vi "MFC.vi"() -> ()   [LabVIEW 2016]
uses:
  controls/UI Data.ctl
  Settings/Settings.ctl
  Logging/Logging Configuration.ctl
  Acquisition/Hardware Configuration.ctl
  controls/UI State.ctl
  support/Message Queue/Enqueue Message (Single).vi
  support/Message Queue/Enqueue Message (Array).vi
  <vilib>/Utility/error.llb/Error Cluster From Error Code.vi
  <vilib>/ErrorRing/Error Ring.xnode
  Settings/Settings.lvlib
  support/Message Queue/Message Queue.lvlib
  Settings/Settings Dialog.vi
  support/User Event - Stop/User Event - Stop.lvlib
  Logging/Logging.lvlib
  Acquisition/Acquisition.lvlib
panel:
  in  "Reset":bool
  out "Total":dbl
  out "R.P":dbl
  in  "S.P.":dbl
  in  "Control":enum32{"1", "2", "4"}(radio)
  in  "Control Mode":T1(radio)
  out "Data":waveform(dbl)[](graph)
  out "2":dbl(knob) caption="总流量" scale=0.0..100.0
  out "流量设定":cluster{dbl, dbl}(knob) scale=0.0..1.0
  in  "Exit":bool
  in  "Stop":bool
  in  "Settings":bool
  in  "Start":bool
  in  "Show Mode":T1(radio)
  out "Status":string
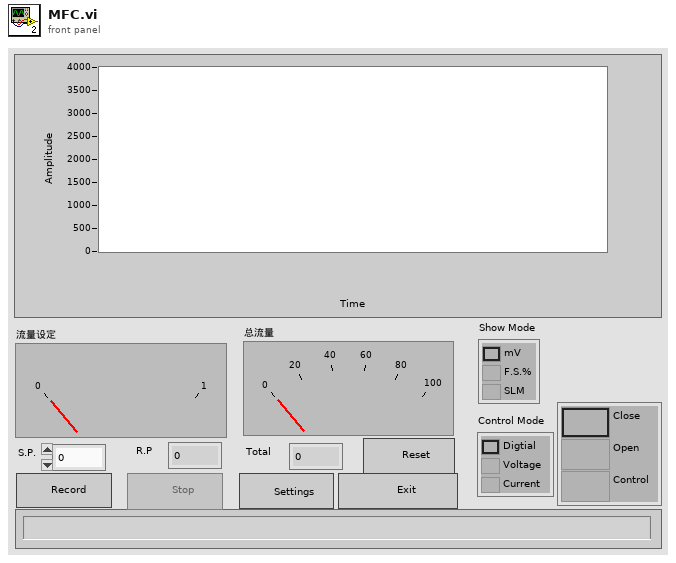
[diagram p1: front panel]
types:
  T1 = enum32{"Radio Selection 1", "Radio Selection 2", "Radio Selection 3"}
  T2 = typedef "UI State.ctl" = enum16{"Idle", "Acquiring and Logging", "Waiting for Exit", "Waiting for Exit (Acq Stopped)", "Waiting for Exit (Log Stopped)", "Waiting for Stop", "Waiting for Stop (Acq Stopped)", "Waiting for Stop (Log Stopped)"}
  T3 = typedef "Settings.lvlib/Settings.ctl" = cluster{"Logging Configuration":T4, "Hardware Config":cluster{"Bautrate":string, "VISA":T5}, "Advance Setting":cluster{"PWM_Step":dbl, "PWM_MIN":dbl, "PWM_MAX":dbl, "DeadZone(mv)":dbl, "SamCycle(ms)":dbl, "Bang-BangTerm":dbl, "ecS":dbl, "ecM":dbl, "ecL":dbl, "eS":dbl, "eM":dbl, "eL":dbl, "Kd F":dbl, "Ki F":dbl, "Kp F":dbl, "Kd":dbl, "Ki":dbl, "Kp":dbl}, "FuzzyMap":cluster{"Table":string[][]}, "ControlMode":cluster{"Control":enum32{"1", "2", "4"}}}
  T4 = typedef "Logging.lvlib/Logging Configuration.ctl" = cluster{"Log File Base Path":path, "save file":bool, "refnum out":refnum<file>}
  T5 = typedef "Acquisition.lvlib/Hardware Configuration.ctl" = refnum<visa-resource-name>
  T6 = typedef "UI Data.ctl" = cluster{"Start Ref":refnum<vi>, "Stop Ref":refnum<vi>, "Settings Ref":refnum<vi>, "Exit Ref":refnum<vi>, "Status Ref":refnum<vi>, "Data Ref":refnum<vi>}
  T7 = typedef "Message Queue.lvlib/All Message Queues.ctl" = cluster{"UI":refnum<queue>, "Acquisition":refnum<queue>, "Logging":refnum<queue>}
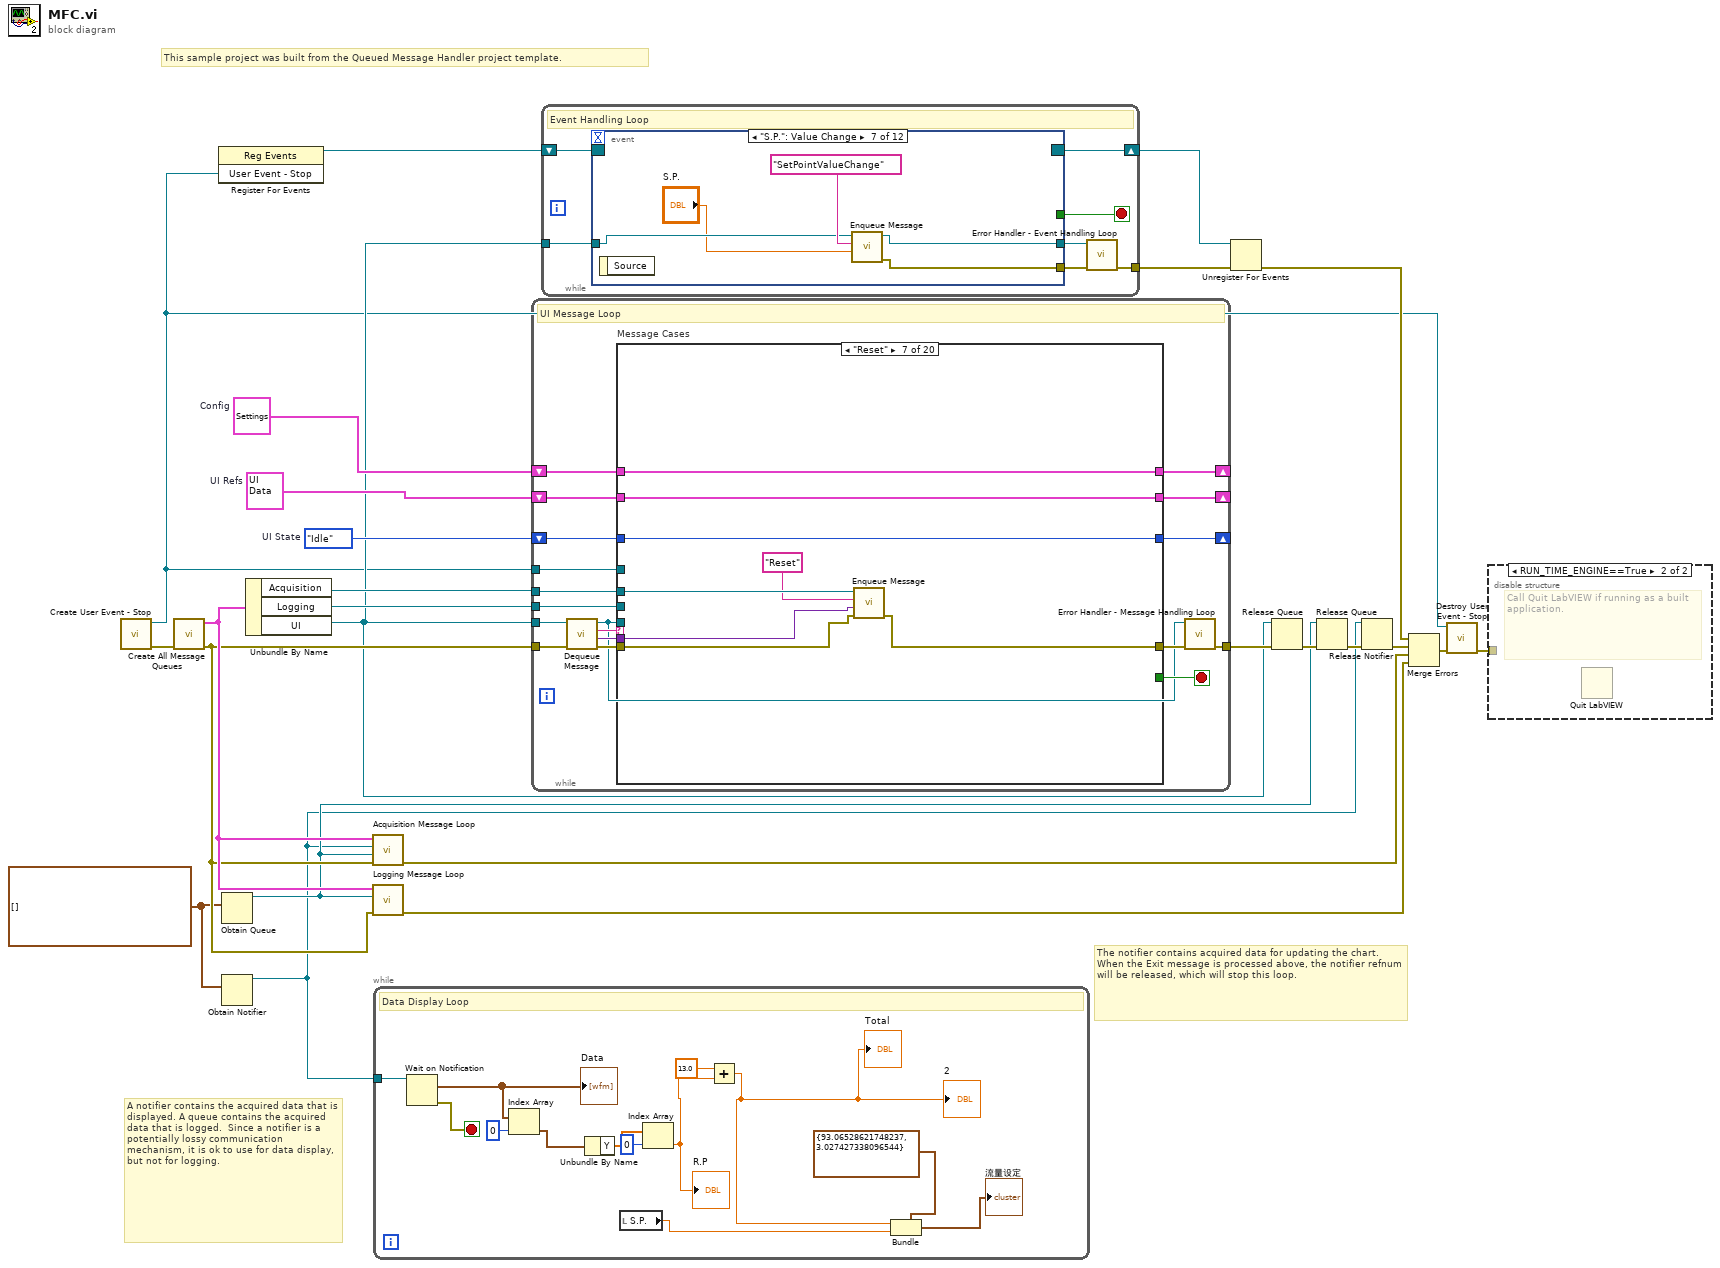
[diagram p0: block diagram]
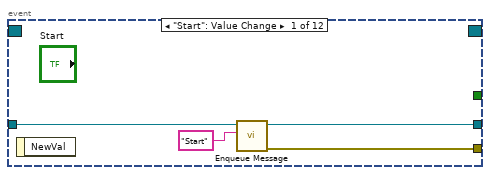
[diagram p3: hidden frame]
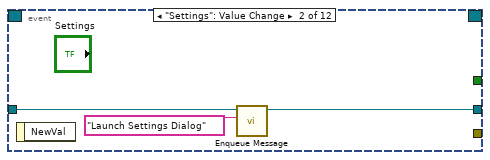
[diagram p4: hidden frame]
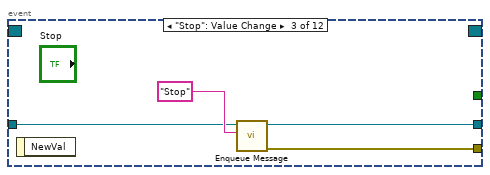
[diagram p5: hidden frame]
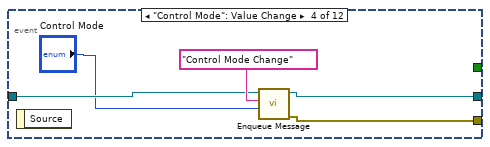
[diagram p6: hidden frame]
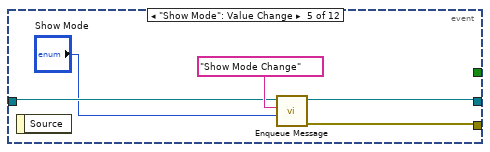
[diagram p7: hidden frame]
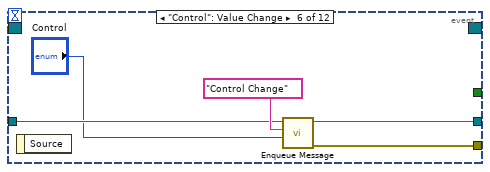
[diagram p8: hidden frame]
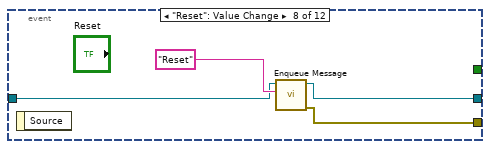
[diagram p9: hidden frame]
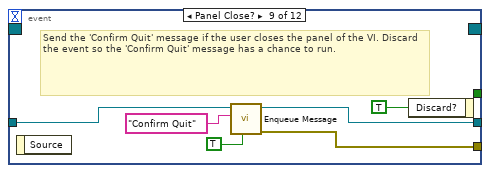
[diagram p10: hidden frame]
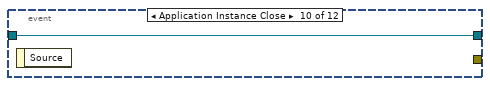
[diagram p11: hidden frame]
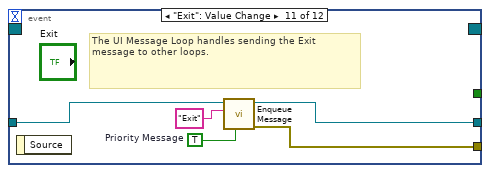
[diagram p12: hidden frame]
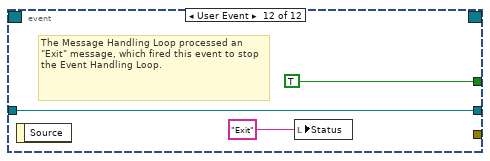
[diagram p13: hidden frame]
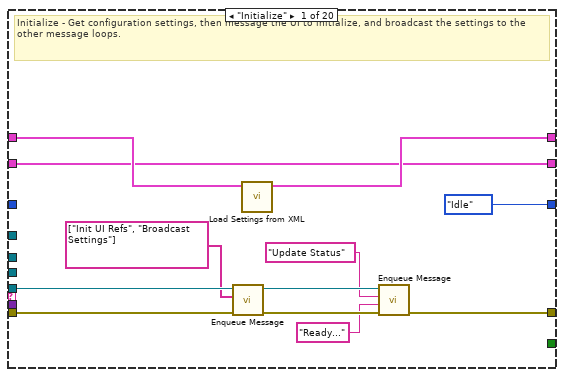
[diagram p14: hidden frame]
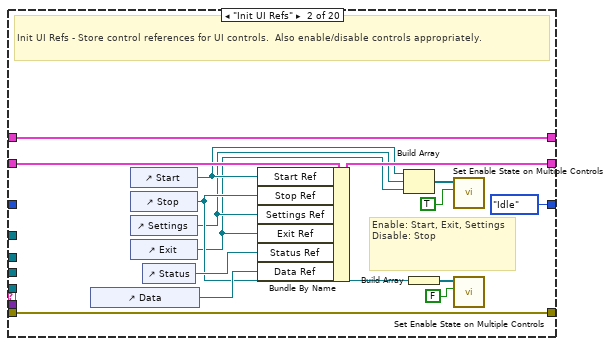
[diagram p15: hidden frame]
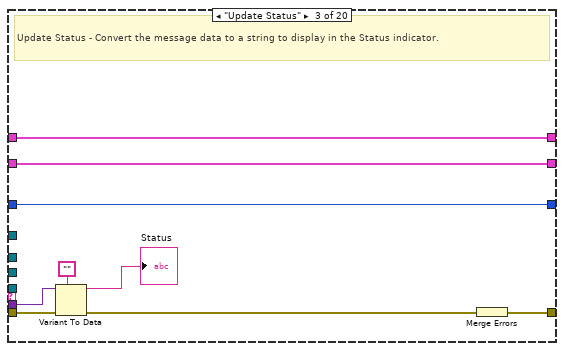
[diagram p16: hidden frame]
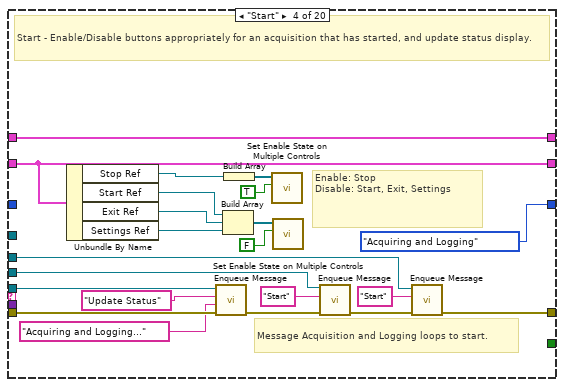
[diagram p17: hidden frame]
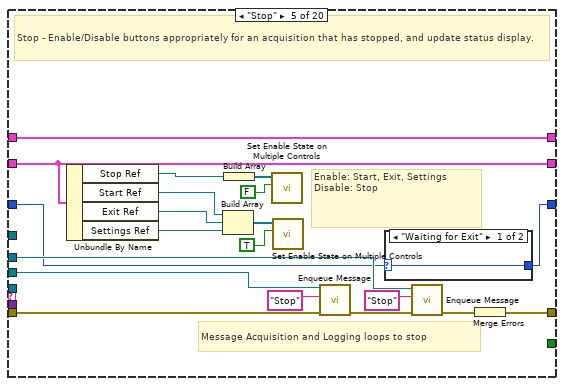
[diagram p18: hidden frame]
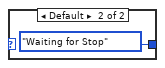
[diagram p19: hidden frame]
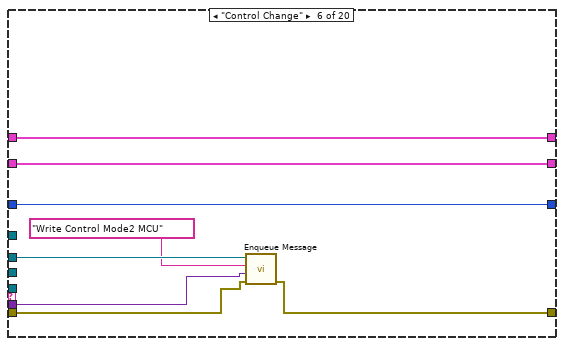
[diagram p20: hidden frame]
diagram:
  w12 = UI_State."Idle"  # UI State
  w3 = waveform(dbl)[] []
  w18 = T3 {"Logging Configuration"={"Log File Base Path"=path "", "save file"=FALSE, "refnum out"=refnum}, "Hardware Config"={"Bautrate"="", "VISA"=""}, "Advance Setting"={"PWM_Step"=0.0, "PWM_MIN"=0.0, "PWM_MAX"=0.0, "DeadZone(mv)"=0.0, "SamCycle(ms)"=0.0, "Bang-BangTerm"=0.0, "ecS"=0.0, "ecM"=0.0, "ecL"=0.0, "eS"=0.0, "eM"=0.0, "eL"=0.0, "Kd F"=0.0, "Ki F"=0.0, "Kp F"=0.0, "Kd"=0.0, "Ki"=0.0, "Kp"=0.0}, "FuzzyMap"={"Table"=[]}, "ControlMode"={"Control"=enum."1"}}  # Config
  w15 = T6 {"Start Ref"=refnum, "Stop Ref"=refnum, "Settings Ref"=refnum, "Exit Ref"=refnum, "Status Ref"=refnum, "Data Ref"=refnum}  # UI Refs
  # "This sample project was built from the Queued Message Handler project template."
  # "A notifier contains the acquired data that is displayed. A queue contains the acquired data that is logged.  Since a notifier is a potentially lossy communication mechanism, it is ok to use for data display, but not for logging."
  # "The notifier contains acquired data for updating the chart. When the Exit message is processed above, the notifier refnum will be released, which will stop this loop."
  n1 = call "Create User Event - Stop.vi"() -> ("error out"=w22:errorcluster, "User Event - Stop"=w1:refnum<user-event>)  [unwired: 10 in]
  n2 = call "Create All Message Queues.vi"("error in (no error)"=w22) -> ("error out"=w19:errorcluster, "Message Queues out"=w21:T7)  [unwired: 9 in]
  n3 = register-events(w1) -> (reference out=w2:refnum<event-registration>)  [unwired: 2 in, 1 out]
  n4 = Obtain Queue(element data type=w3) -> (queue out=w5:refnum<queue>)  [unwired: 4 in, 2 out]
  n5 = Obtain Notifier(notification data type=w3) -> (notifier out=w4:refnum<notifier>)  [unwired: 3 in, 2 out]
  n6 = Unbundle By Name(w21) -> ("Acquisition"=w14:refnum<queue>, "Logging"=w13:refnum<queue>, "UI"=w10:refnum<queue>)
  n7 = call "Acquisition Message Loop.vi"("error in (no error)"=w19, "Data Queue"=w5, "Data Notifier"=w4, "Message Queues"=w21) -> ("error out"=w23:errorcluster)  [unwired: 7 in]
  n8 = call "Logging Message Loop.vi"("error in (no error)"=w19, "Data Queue"=w5, "Message Queues"=w21) -> ("error out"=w20:errorcluster)  [unwired: 8 in]
  n9 = while "Data Display Loop" {
    tunnel: w4 -> [w38]
    stop <- w37 stop-if-true
    # "Data Display Loop"
    n10 = Wait on Notification(notifier=w38) -> (notification=w36:waveform(dbl)[], error out=w37:errorcluster)  [unwired: 3 in, 2 out]
    "Data" <- w36
    n11 = Index Array(array=w36, index=0) -> (element=w34:waveform(dbl))
    n12 = Unbundle By Name(w34) -> ("Y"=w33:dbl[])
    n13 = local read "S.P."() -> (w29:dbl)
    n14 = Index Array(array=w33, index=0) -> (element=w28:dbl)
    "R.P" <- w28
    n15 = Add(x=13.0, y=w28) -> (x+y=w27:dbl)
    "2" <- w27
    "Total" <- w27
    n16 = Bundle(cluster=cluster{dbl, dbl} {93.06528621748237, 3.027427338096544} ("Meter"), w27, w29) -> (→"流量设定":cluster{dbl, dbl})
  }
  n17 = while {
    tunnel: w10 -> [w50]
    tunnel: w1 -> [w55]
    shift-right: [w49] -> _
    shift-left: w18 -> [w48]
    shift-right: [w46] -> _
    shift-left: w15 -> [w47]
    tunnel: w14 -> [w45]
    tunnel: w13 -> [w44]
    shift-right: [w39] -> _
    shift-left: w12 -> [w40]
    tunnel: w19 -> [w54]
    tunnel: [w43] -> w25
    stop <- w56 stop-if-true
    # "UI Message Loop"
    n18 = call "Dequeue Message.vi"("error in (no error)"=w54, "Message Queue"=w50) -> ("error out"=w53:errorcluster, "Message Data"=w51:variant, "Message"=w52:string, "dup Message Queue"=w41:refnum<queue>)  [unwired: 6 in]
    n19 = case "Message Cases" shown="\"Reset\"" w52 {
      selector: w52 -> [_ _ _ _ _ _ _ _ _ _ _ _ _ _ _ _ _ _ _ w320]
      tunnel: w41 -> [w60 _ _ w114 _ _ _ _ _ _ w171 w196 _ _ _ _ w273 _ _ _]
      tunnel: w53 -> [w59 w83 w91 w113 w133 w139 w147 w155 w164 w168 w172 w197 w225 w236 w259 w261 w272 w301 w318 _]
      tunnel: [w64 w83 w92 w96 w134 w138 w146 w154 w164 w168 w169 w194 w229 w237 w257 w264 w271 w311 w317 w319] -> w42
      tunnel: [_ _ _ _ _ _ _ _ _ _ _ _ _ _ _ _ _ TRUE _ _] -> w56
      tunnel: w51 -> [_ _ w90 _ _ w140 w148 w156 _ _ _ _ _ _ w258 w265 _ w299 _ _]
      tunnel: w55 -> [_ _ _ _ _ _ _ _ _ _ _ _ _ _ _ _ _ w312 _ _]
      tunnel: [w67 w82 w86 w112 w132 w144 w152 w160 w163 w167 w175 w200 w219 w230 w253 w269 w276 w310 w316 w323] -> w49
      tunnel: w48 -> [w68 w82 w86 w112 w132 w144 w152 w160 w163 w167 w175 w200 w219 w235 w254 w269 w276 w310 w316 w323]
      tunnel: w47 -> [w61 w81 w85 w109 w131 w143 w151 w159 w162 w166 w174 w199 w223 w239 w260 w268 w275 w309 w315 w322]
      tunnel: [w61 w78 w85 w109 w131 w143 w151 w159 w162 w166 w174 w199 w223 w239 w260 w268 w275 w309 w315 w322] -> w46
      tunnel: w45 -> [_ _ _ w95 w118 w141 w149 w157 _ _ _ _ w222 w231 _ _ _ w308 _ _]
      tunnel: w44 -> [_ _ _ w98 w121 _ _ _ _ _ _ _ w221 _ _ _ _ w307 _ _]
      tunnel: w40 -> [_ _ w84 _ w115 w142 w150 w158 w161 w165 w173 w198 w220 w238 w256 w263 w274 _ w314 w321]
      tunnel: [UI_State."Idle" ("UI State") UI_State."Idle" ("UI State") w84 UI_State."Acquiring and Logging" ("UI State") w116 w142 w150 w158 w161 w165 w170 w195 w220 w238 w256 w263 w270 UI_State."Idle" ("UI State") w314 w321] -> w39
      frame "Initialize" {
        # "Initialize - Get configuration settings, then message the UI to initialize, and broadcast the settings to the other message loops."
        n20 = call-poly "Enqueue Message.vi"("error in (no error)"=w59, "Message Array"=string[] ["Init UI Refs", "Broadcast Settings"], "Message Queue"=w60) -> ("error out"=w66:errorcluster, "dup Message Queue"=w65:refnum<queue>)  [unwired: 7 in]
        n21 = call "Load Settings from XML.vi"("Settings in"=w68) -> ("Settings out"=w67:T3)  [unwired: 9 in, 1 out]
        n22 = call-poly "Enqueue Message.vi"("error in (no error)"=w66, "Message Data"="Ready..." ("Ready..."), "Message"="Update Status", "Message Queue"=w65) -> ("error out"=w64:errorcluster)  [unwired: 6 in, 1 out]
      }
      frame "Init UI Refs" {
        # "Enable: Start, Exit, Settings\nDisable: Stop"
        # "Init UI Refs - Store control references for UI controls.  Also enable/disable controls appropriately."
        n23 = control-ref of="Data"() -> (w79:refnum<vi>)
        n24 = control-ref of="Start"() -> (w72:refnum<vi>)
        n25 = control-ref of="Stop"() -> (w73:refnum<vi>)
        n26 = control-ref of="Settings"() -> (w71:refnum<vi>)
        n27 = control-ref of="Exit"() -> (w70:refnum<vi>)
        n28 = control-ref of="Status"() -> (w80:refnum<vi>)
        n29 = Bundle By Name(cluster=w81, "Start Ref"=w72, "Stop Ref"=w73, "Settings Ref"=w71, "Exit Ref"=w70, "Status Ref"=w80, "Data Ref"=w79) -> (w78:T6)
        n30 = Build Array(w72, w71, w70) -> (w76:refnum<vi>[])
        n31 = Build Array(w73) -> (w75:refnum<vi>[])
        n32 = call "Set Enable State on Multiple Controls.vi"("Enable?"=TRUE, "Controls"=w76) -> ()  [unwired: 10 in]
        n33 = call "Set Enable State on Multiple Controls.vi"("Enable?"=FALSE, "Controls"=w75) -> ()  [unwired: 10 in]
      }
      frame "Update Status" {
        # "Update Status - Convert the message data to a string to display in the Status indicator."
        n34 = Variant To Data(error in=w91, type="", Variant=w90) -> (data=→"Status":string, error out=w88:errorcluster)
        n35 = Merge Errors(w88) -> (w92:errorcluster)
      }
      frame "Start" {
        # "Message Acquisition and Logging loops to start."
        # "Enable: Stop\nDisable: Start, Exit, Settings"
        # "Start - Enable/Disable buttons appropriately for an acquisition that has started, and update status display."
        n36 = Unbundle By Name(w109) -> ("Stop Ref"=w104:refnum<vi>, "Start Ref"=w103:refnum<vi>, "Exit Ref"=w102:refnum<vi>, "Settings Ref"=w101:refnum<vi>)
        n37 = call-poly "Enqueue Message.vi"("error in (no error)"=w113, "Message Data"="Acquiring and Logging..." ("Acquiring and Logging..."), "Message"="Update Status", "Message Queue"=w114) -> ("error out"=w100:errorcluster)  [unwired: 6 in, 1 out]
        n38 = Build Array(w103, w102, w101) -> (w107:refnum<vi>[])
        n39 = Build Array(w104) -> (w106:refnum<vi>[])
        n40 = call "Set Enable State on Multiple Controls.vi"("Enable?"=TRUE, "Controls"=w106) -> ()  [unwired: 10 in]
        n41 = call "Set Enable State on Multiple Controls.vi"("Enable?"=FALSE, "Controls"=w107) -> ()  [unwired: 10 in]
        n42 = call-poly "Enqueue Message.vi"("error in (no error)"=w100, "Message"="Start", "Message Queue"=w98) -> ("error out"=w97:errorcluster)  [unwired: 7 in, 1 out]
        n43 = call-poly "Enqueue Message.vi"("error in (no error)"=w97, "Message"="Start", "Message Queue"=w95) -> ("error out"=w96:errorcluster)  [unwired: 7 in, 1 out]
      }
      frame "Stop" {
        # "Message Acquisition and Logging loops to stop"
        # "Enable: Start, Exit, Settings\nDisable: Stop"
        # "Stop - Enable/Disable buttons appropriately for an acquisition that has stopped, and update status display."
        n44 = Unbundle By Name(w131) -> ("Stop Ref"=w126:refnum<vi>, "Start Ref"=w125:refnum<vi>, "Exit Ref"=w124:refnum<vi>, "Settings Ref"=w123:refnum<vi>)
        n45 = Build Array(w125, w124, w123) -> (w129:refnum<vi>[])
        n46 = Build Array(w126) -> (w128:refnum<vi>[])
        n47 = call "Set Enable State on Multiple Controls.vi"("Enable?"=FALSE, "Controls"=w128) -> ()  [unwired: 10 in]
        n48 = call "Set Enable State on Multiple Controls.vi"("Enable?"=TRUE, "Controls"=w129) -> ()  [unwired: 10 in]
        n49 = call-poly "Enqueue Message.vi"("error in (no error)"=w133, "Message"="Stop", "Message Queue"=w121) -> ("error out"=w120:errorcluster)  [unwired: 7 in, 1 out]
        n50 = case shown="\"Waiting for Exit\"" w115 {
          selector: w115 -> [w135 _]
          tunnel: [w135 UI_State."Waiting for Stop" ("UI State")] -> w116
          frame "Waiting for Exit" {
          }
          frame Default {
          }
        }
        n51 = call-poly "Enqueue Message.vi"("error in (no error)"=w120, "Message"="Stop", "Message Queue"=w118) -> ("error out"=w119:errorcluster)  [unwired: 7 in, 1 out]
        n52 = Merge Errors(w119) -> (w134:errorcluster)
      }
      frame "Control Change" {
        n53 = call-poly "Enqueue Message.vi"("error in (no error)"=w139, "Message Data"=w140, "Message"="Write Control Mode2 MCU", "Message Queue"=w141) -> ("error out"=w138:errorcluster)  [unwired: 6 in, 1 out]
      }
      frame "Reset" {
        n54 = call-poly "Enqueue Message.vi"("error in (no error)"=w147, "Message Data"=w148, "Message"="Reset", "Message Queue"=w149) -> ("error out"=w146:errorcluster)  [unwired: 6 in, 1 out]
      }
      frame "SetPointValueChange" {
        n55 = call-poly "Enqueue Message.vi"("error in (no error)"=w155, "Message Data"=w156, "Message"="SetPointValueChange", "Message Queue"=w157) -> ("error out"=w154:errorcluster)  [unwired: 6 in, 1 out]
      }
      frame "Control Mode Change" {
      }
      frame "Show Mode Change" {
      }
      frame "Acquisition Stopped" {
        # "Logic for determining what action to take when the acquisition has stopped."
        n56 = case shown="\"Waiting for Exit (Log Stopped)\"" w173 {
          selector: w173 -> [w177 _ _ _ _]
          tunnel: w172 -> [w176 w179 w181 w187 w193]
          tunnel: w171 -> [_ _ _ w185 w190]
          tunnel: [w177 UI_State."Waiting for Exit (Acq Stopped)" ("UI State") UI_State."Waiting for Stop (Acq Stopped)" ("UI State") UI_State."Idle" ("UI State") UI_State."Idle" ("UI State")] -> w170
          tunnel: [w176 w179 w181 w186 w191] -> w169
          frame Default {
          }
          frame "Waiting for Exit", "Waiting for Exit (Acq Stopped)" {
          }
          frame "Waiting for Stop", "Waiting for Stop (Acq Stopped)" {
          }
          frame "Waiting for Exit (Log Stopped)" {
            # "If we are waiting to exit, and the logging has already stopped, then the \"Acquisition Stopped\" message indicates that it is time to exit."
            n57 = call-poly "Enqueue Message.vi"("Priority Message? (F)"=TRUE, "error in (no error)"=w187, "Message"="Exit", "Message Queue"=w185) -> ("error out"=w186:errorcluster)  [unwired: 6 in, 1 out]
          }
          frame "Waiting for Stop (Log Stopped)" {
            # "If we are waiting to stop, and the logging has already stopped, then the \"Acquisition Stopped\" message indicates that it is time to stop."
            n58 = call-poly "Enqueue Message.vi"("error in (no error)"=w193, "Message Data"="Ready..." ("Ready..."), "Message"="Update Status", "Message Queue"=w190) -> ("error out"=w191:errorcluster)  [unwired: 6 in, 1 out]
          }
        }
      }
      frame "Logging Stopped" {
        # "Logic for determining what action to take when the logging has stopped."
        n59 = case shown="\"Waiting for Stop (Acq Stopped)\"" w198 {
          selector: w198 -> [w202 _ _ _ _]
          tunnel: w197 -> [w201 w204 w206 w212 w215]
          tunnel: w196 -> [_ _ _ w210 w214]
          tunnel: [w202 UI_State."Waiting for Exit (Log Stopped)" ("UI State") UI_State."Waiting for Stop (Log Stopped)" ("UI State") UI_State."Idle" ("UI State") UI_State."Idle" ("UI State")] -> w195
          tunnel: [w201 w204 w206 w211 w213] -> w194
          frame Default {
          }
          frame "Waiting for Exit", "Waiting for Exit (Log Stopped)" {
          }
          frame "Waiting for Stop", "Waiting for Stop (Log Stopped)" {
          }
          frame "Waiting for Exit (Acq Stopped)" {
            # "If we are waiting to exit, and the acquisition has already stopped, then the \"Logging Stopped\" message indicates that it is time to exit."
            n60 = call-poly "Enqueue Message.vi"("Priority Message? (F)"=TRUE, "error in (no error)"=w212, "Message"="Exit", "Message Queue"=w210) -> ("error out"=w211:errorcluster)  [unwired: 6 in, 1 out]
          }
          frame "Waiting for Stop (Acq Stopped)" {
            # "If we are waiting to stop, and the acquisition has already stopped, then the \"Logging Stopped\" message indicates that it is time to stop."
            n61 = call-poly "Enqueue Message.vi"("error in (no error)"=w215, "Message Data"="Ready..." ("Ready..."), "Message"="Update Status", "Message Queue"=w214) -> ("error out"=w213:errorcluster)  [unwired: 6 in, 1 out]
          }
        }
      }
      frame "Broadcast settings" {
        w224 = "Update Settings" ("Message")
        # "Broadcast settings - Send the 'Update Settings' message to the Logging and Acquisition message loops."
        n62 = Unbundle By Name(w219) -> ("Logging Configuration"=w227:T4)
        n63 = call-poly "Enqueue Message.vi"("Message Data"=w219, "Message"=w224, "Message Queue"=w222) -> ("error out"=w228:errorcluster)  [unwired: 7 in, 1 out]
        n64 = call-poly "Enqueue Message.vi"("error in (no error)"=w228, "Message Data"=w227, "Message"=w224, "Message Queue"=w221) -> ("error out"=w226:errorcluster)  [unwired: 6 in, 1 out]
        n65 = Merge Errors(w226, w225) -> (w229:errorcluster)
      }
      frame "Launch Settings Dialog" {
        # "Launch Settings Dialog - Launch the Settings Dialog when the user clicks the 'Settings' button."
        n66 = call-by-ref "?"("Settings in"=w235, "error in (no error)"=w236) -> ("FuzzyMap change?"=w233:bool, "Settings out"=w230:T3, "PID change?"=w234:bool, "error out"=w232:errorcluster)  [unwired: 6 in, 3 out]
        n67 = case shown="True" w234 {
          tunnel: w231 -> [w250 _]
          tunnel: w232 -> [w249 w251]
          tunnel: [w248 w251] -> w237
          tunnel: w230 -> [w246 _]
          frame True {
            n68 = call-poly "Enqueue Message.vi"("error in (no error)"=w249, "Message Data"=w246, "Message"="SavePIDSetting2MCU", "Message Queue"=w250) -> ("error out"=w248:errorcluster)  [unwired: 6 in, 1 out]
          }
          frame False {
          }
        }
        n69 = case shown="True" w233 {
          tunnel: w231 -> [w244 _]
          tunnel: w232 -> [w243 w245]
          tunnel: [w242 w245] -> _
          tunnel: w230 -> [w240 _]
          frame True {
            n70 = call-poly "Enqueue Message.vi"("error in (no error)"=w243, "Message Data"=w240, "Message"="SaveFuzzyMapSetting2MCU", "Message Queue"=w244) -> ("error out"=w242:errorcluster)  [unwired: 6 in, 1 out]
          }
          frame False {
          }
        }
      }
      frame "UpdateHoldingRegs" {
        n71 = Variant To Data(error in=w259, type=w254, Variant=w258) -> (data=w255:T3, error out=w257:errorcluster)
        n72 = Select(t=w254, s=w257, f=w255) -> (s? t:f=w253:T3)
        n73 = Unbundle By Name(w253) -> ("ControlMode.Control"=w252:enum32{"1", "2", "4"})
        n74 = local write "Control"(w252) -> ()
      }
      frame "Error" {
        # "Error - Display an error dialog. This message is sent by the \"Error Handler\" VIs at the end of other loops in this application."
        n75 = Variant To Data(error in=w261, type=errorcluster {"status"=FALSE, "code"=0, "source"=""} ("error constant"), Variant=w265) -> (data=w262:errorcluster, error out=w266:errorcluster)
        n76 = call <vilib>:"Simple Error Handler.vi"("error in (no error)"=w262) -> ()  [unwired: 4 in, 5 out]
        n77 = Merge Errors(w266) -> (w264:errorcluster)
      }
      frame "Confirm Quit" {
        # "Confirm Quit - Message that can confirm whether or not the user wants to exit the application."
        n78 = case shown="\"Acquiring and Logging\"" w274 {
          tunnel: w273 -> [w282 w286]
          tunnel: w272 -> [w281 w285]
          tunnel: [w280 w284] -> w271
          tunnel: [UI_State."Idle" ("UI State") w283] -> w270
          frame Default {
            # "If 'Confirm Quit' comes in while the system is idle, there is no need for a confirmation message."
            n79 = call-poly "Enqueue Message.vi"("Priority Message? (F)"=TRUE, "error in (no error)"=w281, "Message"="Exit", "Message Queue"=w282) -> ("error out"=w280:errorcluster)  [unwired: 6 in, 1 out]
          }
          frame "Acquiring and Logging" {
            n80 = Two Button Dialog(message="Are you sure you want to quit while the acquisition is running?" ("Confirm Quit Message"), 1:"No" ("No"), 2:"Yes" ("Yes")) -> (T button?=w287:bool)
            n81 = case shown="True" w287 {
              tunnel: w286 -> [_ w296]
              tunnel: w285 -> [w292 w297]
              tunnel: [w292 w295] -> w284
              tunnel: [UI_State."Acquiring and Logging" ("UI State") UI_State."Waiting for Exit" ("UI State")] -> w283
              frame False {
                # "User did not want to quit."
              }
              frame True {
                n82 = call-poly "Enqueue Message.vi"("error in (no error)"=w297, "Message"="Stop", "Message Queue"=w296) -> ("error out"=w295:errorcluster)  [unwired: 7 in, 1 out]
              }
            }
          }
        }
      }
      frame "Exit" {
        w303 = TRUE ("Priority Message? (F)")
        w304 = "Exit" ("Message")
        # "Popup an error dialog if 'Exit' was called as a result of an error."
        # "Stop the VI"
        # "Exit - Send Exit messages to the Acquisition and Logging loops, and fire the user event to stop the Event Handling Loop."
        n83 = Variant To Data(type=errorcluster {"status"=FALSE, "code"=0, "source"=""} ("error constant"), Variant=w299) -> (data=w298:errorcluster)  [unwired: 1 in, 1 out]
        n84 = call <vilib>:"Simple Error Handler.vi"("error in (no error)"=w298) -> ()  [unwired: 4 in, 5 out]
        n85 = call-poly "Enqueue Message.vi"("Priority Message? (F)"=w303, "error in (no error)"=w301, "Message"=w304, "Message Queue"=w308) -> ("error out"=w305:errorcluster)  [unwired: 6 in, 1 out]
        n86 = call-poly "Enqueue Message.vi"("Priority Message? (F)"=w303, "error in (no error)"=w305, "Message"=w304, "Message Queue"=w307) -> ("error out"=w302:errorcluster)  [unwired: 6 in, 1 out]
        n87 = call "Fire User Event - Stop.vi"("error in (no error)"=w302, "User Event - Stop"=w312) -> ("error out"=w311:errorcluster)  [unwired: 9 in]
      }
      frame "---Copy This Frame---" {
        # "Duplicate this frame when creating new messages.  Change this comment in the duplicated frame to describe this message."
        n88 = Merge Errors(w318) -> (w317:errorcluster)
      }
      frame Default {
        # "'Default' case only runs if there is a message that isn't defined in any of the other cases.  Output a programming error."
        n89 = xnode "Error Ring"("parameter 0"=w320) -> ("error out"=w319:errorcluster)
      }
    }
    n90 = call "Error Handler - Message Handling Loop.vi"("error in (no error)"=w42, "Message Queue"=w41) -> ("dup error in"=w43:errorcluster)  [unwired: 8 in, 1 out]
  }
  n91 = while {
    tunnel: w10 -> [w336]
    tunnel: [w333] -> w24
    shift-right: [w335] -> w16
    shift-left: w2 -> [w337]
    stop <- w334 stop-if-true
    # "Event Handling Loop"
    n92 = event shown="[6] \"S.P.\": Value Change" {
      selector: w337 -> [_ _ _ _ _ _ _ _ _ _ _ _]
      dyn-events: [_ _ _ _ _ _ _ _ _ _ _ _] -> w335
      timeout: _ -> [_ _ _ _ _ _ _ _ _ _ _ _]
      tunnel: [_ _ _ _ _ _ _ _ _ _ _ TRUE ("Discard?")] -> w334
      tunnel: w336 -> [w341 w343 w347 w351 w355 w360 w367 w371 w376 w379 w381 w385]
      tunnel: [w339 _ w346 w352 w357 w362 w365 w369 w374 _ w384 _] -> w332
      tunnel: [w338 w342 w345 w350 w356 w361 w366 w370 w375 w379 w380 w385] -> w331
      event "Start": Value Change {
        n93 = event-data() -> ()  [unwired: 1 in, 1 out]
        n94 = call-poly "Enqueue Message.vi"("Message"="Start", "Message Queue"=w341) -> ("error out"=w339:errorcluster, "dup Message Queue"=w338:refnum<queue>)  [unwired: 8 in]
      }
      event "Settings": Value Change {
        n95 = event-data() -> ()  [unwired: 1 in, 1 out]
        n96 = call-poly "Enqueue Message.vi"("Message"="Launch Settings Dialog", "Message Queue"=w343) -> ("dup Message Queue"=w342:refnum<queue>)  [unwired: 8 in, 1 out]
      }
      event "Stop": Value Change {
        n97 = event-data() -> ()  [unwired: 1 in, 1 out]
        n98 = call-poly "Enqueue Message.vi"("Message"="Stop", "Message Queue"=w347) -> ("error out"=w346:errorcluster, "dup Message Queue"=w345:refnum<queue>)  [unwired: 8 in]
      }
      event "Control Mode": Value Change {
        n99 = event-data() -> ()  [unwired: 1 in, 1 out]
        n100 = call-poly "Enqueue Message.vi"("Message Data"="Control Mode", "Message"="Control Mode Change", "Message Queue"=w351) -> ("error out"=w352:errorcluster, "dup Message Queue"=w350:refnum<queue>)  [unwired: 7 in]
      }
      event "Show Mode": Value Change {
        n101 = event-data() -> ()  [unwired: 1 in, 1 out]
        n102 = call-poly "Enqueue Message.vi"("Message Data"="Show Mode", "Message"="Show Mode Change", "Message Queue"=w355) -> ("error out"=w357:errorcluster, "dup Message Queue"=w356:refnum<queue>)  [unwired: 7 in]
      }
      event "Control": Value Change {
        n103 = event-data() -> ()  [unwired: 1 in, 1 out]
        n104 = call-poly "Enqueue Message.vi"("Message Data"="Control", "Message"="Control Change", "Message Queue"=w360) -> ("error out"=w362:errorcluster, "dup Message Queue"=w361:refnum<queue>)  [unwired: 7 in]
      }
      event "S.P.": Value Change {
        n105 = event-data() -> ()  [unwired: 1 in, 1 out]
        n106 = call-poly "Enqueue Message.vi"("Message Data"="S.P.", "Message"="SetPointValueChange", "Message Queue"=w367) -> ("error out"=w365:errorcluster, "dup Message Queue"=w366:refnum<queue>)  [unwired: 7 in]
      }
      event "Reset": Value Change {
        n107 = event-data() -> ()  [unwired: 1 in, 1 out]
        n108 = call-poly "Enqueue Message.vi"("Message"="Reset", "Message Queue"=w371) -> ("error out"=w369:errorcluster, "dup Message Queue"=w370:refnum<queue>)  [unwired: 8 in]
      }
      event Panel Close? {
        # "Send the 'Confirm Quit' message if the user closes the panel of the VI. Discard the event so the 'Confirm Quit' message has a chance to run."
        n109 = event-data() -> ()  [unwired: 1 in, 1 out]
        n110 = call-poly "Enqueue Message.vi"("Priority Message? (F)"=TRUE, "Message"="Confirm Quit", "Message Queue"=w376) -> ("error out"=w374:errorcluster, "dup Message Queue"=w375:refnum<queue>)  [unwired: 7 in]
        n111 = event-data("Discard?"=TRUE) -> ()  [unwired: 1 in, 1 out]
      }
      event Application Instance Close {
        n112 = event-data() -> ()  [unwired: 1 in, 1 out]
      }
      event "Exit": Value Change {
        w382 = TRUE  # Priority Message
        # "The UI Message Loop handles sending the Exit message to other loops."
        n113 = event-data() -> ()  [unwired: 1 in, 1 out]
        n114 = call-poly "Enqueue Message.vi"("Priority Message? (F)"=w382, "Message"="Exit", "Message Queue"=w381) -> ("error out"=w384:errorcluster, "dup Message Queue"=w380:refnum<queue>)  [unwired: 7 in]
      }
      event User Event {
        # "The Message Handling Loop processed an \"Exit\" message, which fired this event to stop the Event Handling Loop."
        n115 = event-data() -> ()  [unwired: 1 in, 1 out]
        n116 = local write "Status"("Exit" ("Exit String")) -> ()
      }
    }
    n117 = call "Error Handler - Event Handling Loop.vi"("error in (no error)"=w332, "Message Queue"=w331) -> ("dup error in"=w333:errorcluster)  [unwired: 8 in, 1 out]
  }
  n118 = Unregister For Events(event registration refnum=w16, error in=w24) -> (error out=w17:errorcluster)
  n119 = Release Queue(queue=w10, error in (no error)=w25) -> (error out=w8:errorcluster)  [unwired: 1 in, 2 out]
  n120 = Release Queue(queue=w5, error in (no error)=w8) -> (error out=w7:errorcluster)  [unwired: 1 in, 2 out]
  n121 = Release Notifier(notifier=w4, error in (no error)=w7) -> (error out=w6:errorcluster)  [unwired: 1 in, 2 out]
  n122 = Merge Errors(w17, w6, w23, w20) -> (w11:errorcluster)
  n123 = call "Destroy User Event - Stop.vi"("error in (no error)"=w11, "User Event - Stop"=w1) -> ("error out"=w9:errorcluster)  [unwired: 9 in]
  n124 = disable-structure shown="RUN_TIME_ENGINE==True" {
    disable-tunnel: w9 -> [_ _]
    frame condition #0 (active) {
    }
    frame condition #1 {
      # "Call Quit LabVIEW if running as a built application."
      n125 = Quit LabVIEW() -> ()  [unwired: 1 in]
    }
  }
